vi "GEOM_ReadCoordsReference.vi"(6 "Database RefNum in":T1, 8 "error in (no error)":errorcluster, 9 "detrows":u32, 10 "detcols":u32, 11 "file path":path) -> (0 "error out":errorcluster, 2 "ref":T2, 3 "file path out":path)   [LabVIEW 2016]
uses:
  GEOM_CoordsRef.ctl
  DBSHAND/private/vis/DatabaseHand_RefNum.ctl
  GEOM_VAR_action.ctl
  <vilib>/Utility/config.llb/Read Key (String).vi
  DBSHAND/private/vis/DatabaseHand_Element_Set(U32).vi
  DBSHAND/private/vis/DatabaseHand_Element_Set(string).vi
  <vilib>/Utility/config.llb/NI_LVConfig.lvlib
panel:
  in  "GEOM_coordsref":T2
  in  "section":string="COORDSORIG"
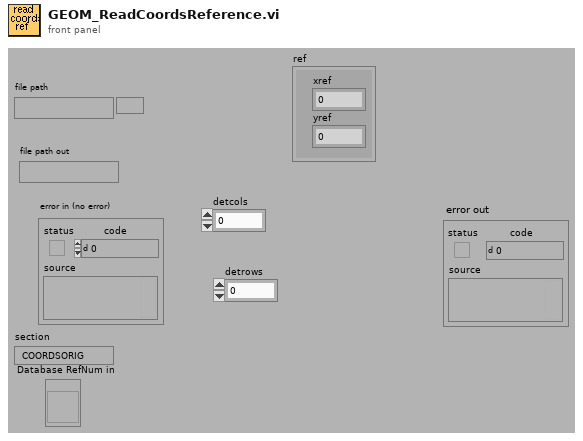
[diagram p1: front panel]
types:
  T1 = typedef "DatabaseHand_RefNum.ctl" = refnum<vi>
  T2 = typedef "GEOM_CoordsRef.ctl" = cluster{"xref":u32, "yref":u32}
  T3 = typedef "GEOM_VAR_action.ctl" = enum16{"read", "write"}
  T4 = typedef "NI_LVConfig.lvlib/Config Data RefNum.ctl" = refnum<k1>
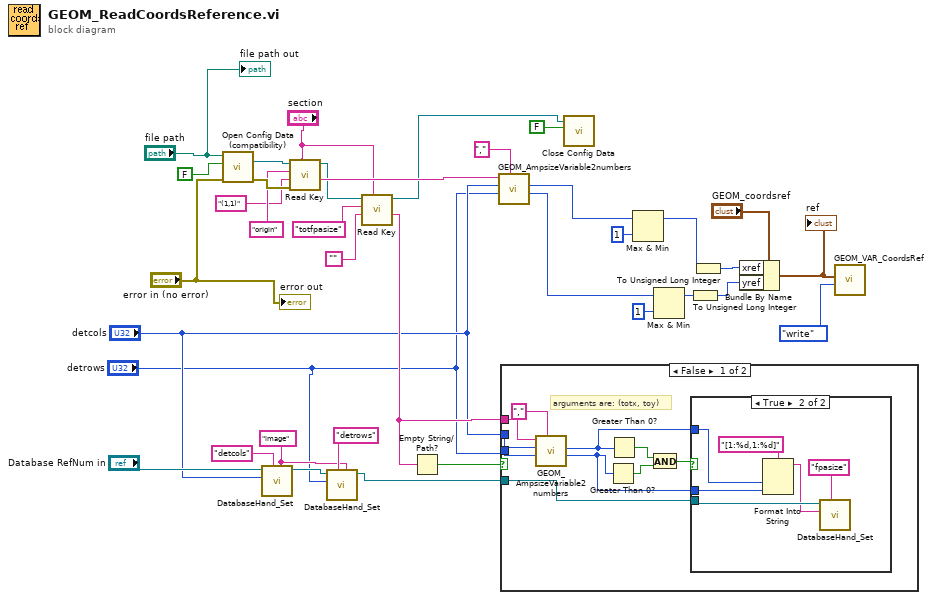
[diagram p0: block diagram]
diagram:
  w6 = "image" ("group")
  n1 = call <vilib>:"Open Config Data (compatibility).vi"("error in (no error)"="error in (no error)", "create file if necessary (T)"=FALSE ("create file if necessary? (T)"), "configuration file path"="file path") -> ("error out"=w33:errorcluster, "refnum"=w32:T4)  [unwired: 6 in, 1 out]
  n2 = call-poly "DatabaseHand_Set.vi"("group"=w6, "name"="detcols", "value"="detcols", "Database RefNum in"="Database RefNum in") -> ("Database RefNum out"=w8:T1)  [unwired: 4 in, 3 out]
  n3 = call-poly <vilib>:"Read Key.vi"("section"="section", "error in (no error)"=w33, "default value"="(1,1)" ("key"), "key"="origin", "refnum"=w32) -> ("value"=w20:string, "refnum out"=w16:T4)  [unwired: 1 in, 4 out]
  n4 = call-poly "DatabaseHand_Set.vi"("group"=w6, "name"="detrows", "value"="detrows", "Database RefNum in"=w8) -> ("Database RefNum out"=w4:T1)  [unwired: 4 in, 3 out]
  n5 = call-poly <vilib>:"Read Key.vi"("section"="section", "default value"="", "key"="totfpasize", "refnum"=w16) -> ("value"=w10:string, "refnum out"=w15:T4)  [unwired: 2 in, 4 out]
  n6 = Empty String/Path?(string/path=w10) -> (empty?=w11:bool)
  n7 = call "GEOM_AmpsizeVariable2numbers.vi"("separator"=",", "detrows"="detrows", "detcols"="detcols", "ampval"=w20) -> ("amprows"=w19:i32, "ampcols"=w21:i32)  [unwired: 6 out]
  n8 = case shown="False" w11 {
    tunnel: w10 -> [w46 _]
    tunnel: "detcols" -> [w43 _]
    tunnel: "detrows" -> [w42 _]
    tunnel: w4 -> [w38 _]
    frame False {
      # "arguments are: (totx, toy)"
      n9 = call "GEOM_AmpsizeVariable2numbers.vi"("separator"=",", "detrows"=w42, "detcols"=w43, "ampval"=w46) -> ("amprows"=w39:i32, "ampcols"=w40:i32)  [unwired: 6 out]
      n10 = Greater Than 0?(x=w39) -> (x > 0?=w44:bool)
      n11 = Greater Than 0?(x=w40) -> (x > 0?=w45:bool)
      n12 = And(x=w45, y=w44) -> (x .and. y?=w41:bool)
      n13 = case shown="True" w41 {
        tunnel: w38 -> [_ w51]
        tunnel: w40 -> [_ w49]
        tunnel: w39 -> [_ w48]
        frame False {
        }
        frame True {
          n14 = Format Into String(format string="[1:%d,1:%d]", w49, w48) -> (resulting string=w47:string)  [unwired: 2 in, 1 out]
          n15 = call-poly "DatabaseHand_Set.vi"("name"="fpasize", "value"=w47, "Database RefNum in"=w51) -> ()  [unwired: 5 in, 4 out]
        }
      }
    }
    frame True {
    }
  }
  n16 = call <vilib>:"Close Config Data.vi"("write file if changed (T)"=FALSE ("write configuration file? (F)"), "refnum"=w15) -> ()  [unwired: 1 in, 9 out]
  n17 = Max & Min(x=w21, y=1) -> (max(x,y)=w26:i32)  [unwired: 1 out]
  n18 = Max & Min(x=w19, y=1) -> (max(x,y)=w17:i32)  [unwired: 1 out]
  n19 = To Unsigned Long Integer(number=w17) -> (unsigned 32bit integer=w24:u32)
  n20 = To Unsigned Long Integer(number=w26) -> (unsigned 32bit integer=w25:u32)
  n21 = Bundle By Name(cluster="GEOM_coordsref", "xref"=w25, "yref"=w24) -> (w29:T2)
  "ref" <- w29
  n22 = call "GEOM_VAR_CoordsRef.vi"("Action"=GEOM_VAR_action."write", "GEOM_coordsref"=w29) -> ()  [unwired: 10 out]
  "file path out" <- "file path"
  "error out" <- "error in (no error)"
